vi "Task6.vi"() -> ()   [LabVIEW 2017]
panel:
  out "Waveform Chart":u32(graph)
  in  "stop":bool
  out "Numeric":u8
  in  "8bit switches":bool[](array[boolean])
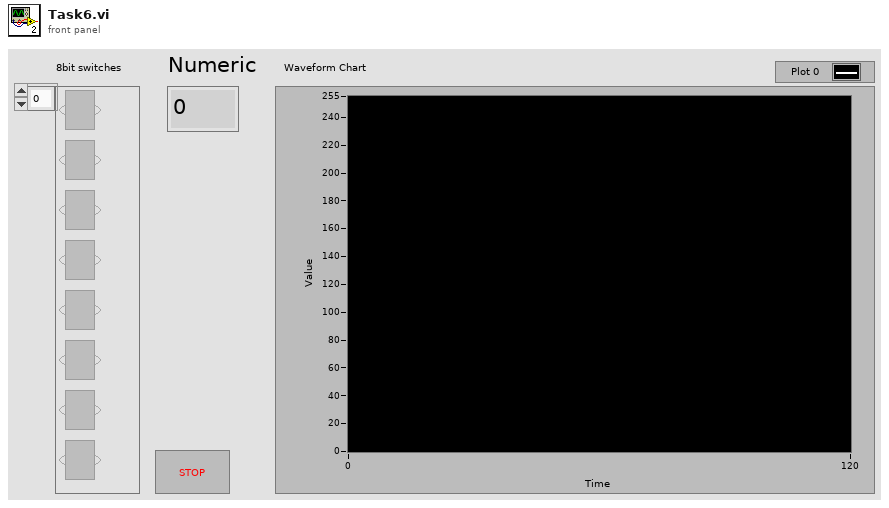
[diagram p1: front panel]
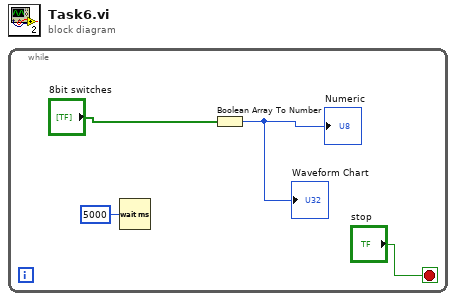
[diagram p0: block diagram]
diagram:
  n1 = while {
    stop <- "stop" stop-if-true
    n2 = Wait (ms)(milliseconds to wait=u32 5000) -> ()  [unwired: 1 out]
    n3 = Boolean Array To Number(Boolean array="8bit switches") -> (number=→"Numeric" →"Waveform Chart":u32)
  }
